vi "getAnalyisNuber.vi"(8 "Erreur en entrée":errorcluster caption="entrée d'erreur (pas d'erreur)", 9 "Nom de l'analyse en entrée":string, 11 "VISA resource en entrée":refnum<visa-resource-name>) -> (0 "error out":errorcluster caption="sortie d'erreur", 1 "Nom de l'analyse en sortie":string, 2 "Numéro de la\nprochaine analyse":i32, 3 "VISA resource en sortie":refnum<visa-resource-name>)   [LabVIEW 2019]
panel:
  out "Tableau":string[](array[string])
  out "Nom des fichiers":string[](array[string])
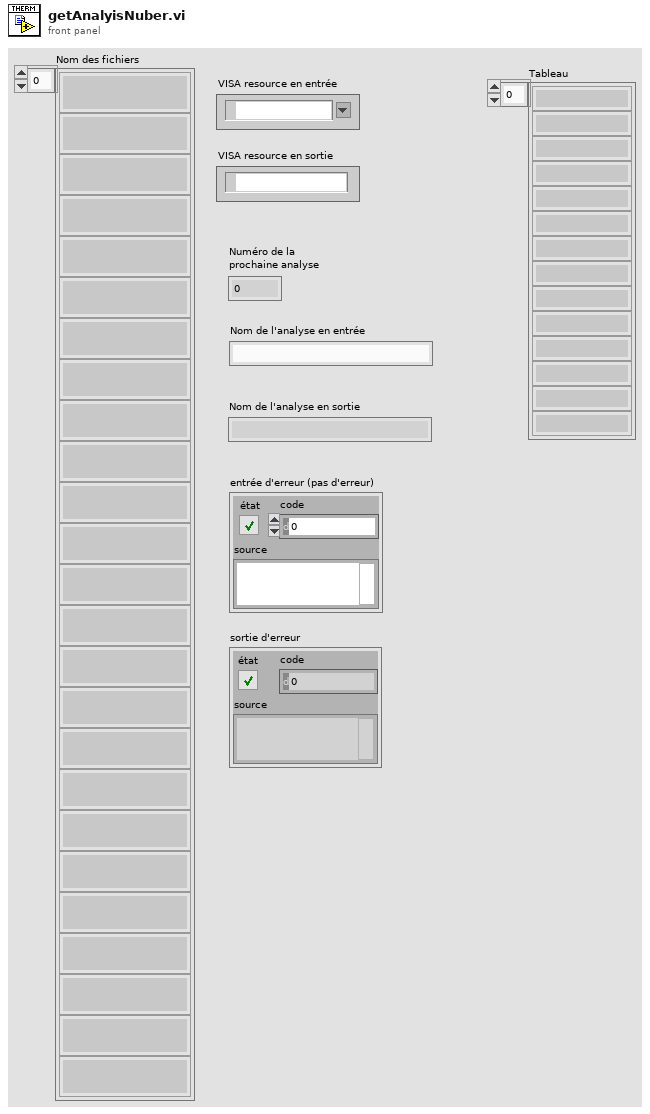
[diagram p1: front panel]
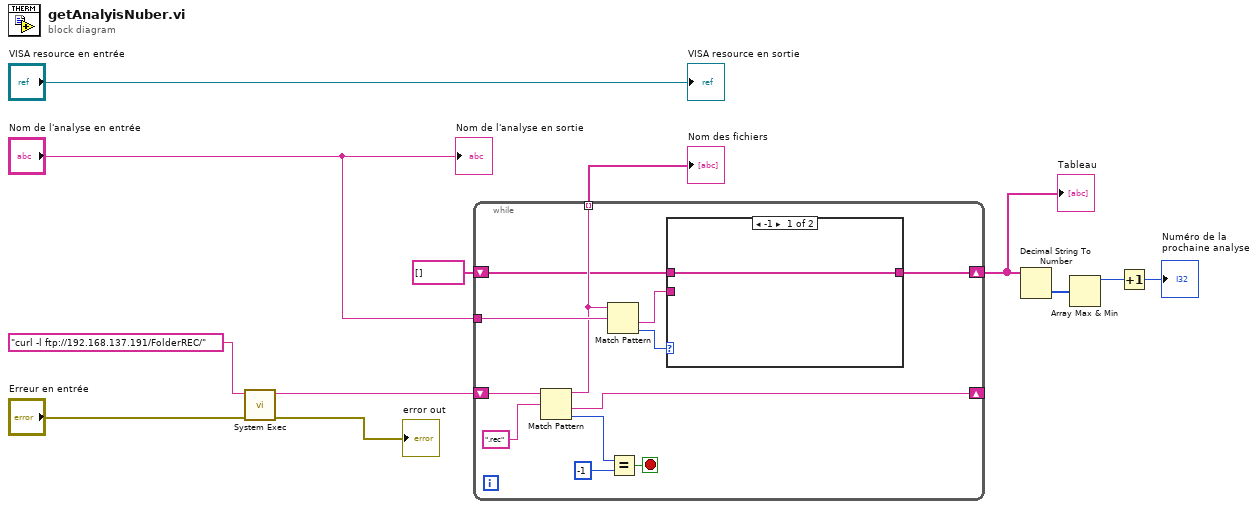
[diagram p0: block diagram]
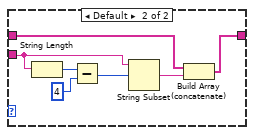
[diagram p2: hidden frame]
diagram:
  n1 = call <vilib>:"System Exec.vi"("error in (no error)"="Erreur en entrée", "command line"="curl -l ftp://192.168.137.191/FolderREC/") -> ("error out"=→"error out":errorcluster, "standard output"=w10:string)  [unwired: 6 in, 2 out]
  n2 = while {
    shift-right: [w20] -> _
    shift-left: w10 -> [w24]
    tunnel: [w18] -> w7 mode=indexing
    tunnel: "Nom de l'analyse en entrée" -> [w19]
    shift-right: [w17] -> w6
    shift-left: string[] [] -> [w16]
    stop <- w21 stop-if-true
    n3 = Match Pattern(string=w24, regular expression=".rec" ("expression régulière")) -> (before substring=w18:string, after substring=w20:string, offset past match=w23:i32)  [unwired: 1 in, 1 out]
    n4 = Match Pattern(string=w18, regular expression=w19) -> (after substring=w14:string, offset past match=w15:i32)  [unwired: 1 in, 2 out]
    n5 = Equal?(x=w23, y=-1) -> (x = y?=w21:bool)
    n6 = case shown="-1" w15 {
      tunnel: [w25 w32] -> w17
      tunnel: w14 -> [_ w27]
      tunnel: w16 -> [w25 w31]
      frame -1 {
      }
      frame Default {
        n7 = String Length(string=w27) -> (length=w29:i32)
        n8 = Subtract(x=w29, y=4) -> (x-y=w30:i32)
        n9 = String Subset(string=w27, offset (0)=w30) -> (substring=w26:string)  [unwired: 1 in]
        n10 = Build Array (concatenate)(w31, w26) -> (w32:string[])
      }
    }
  }
  "Nom des fichiers" <- w7
  "Tableau" <- w6
  n11 = Decimal String To Number(string=w6) -> (number=w5:i32[])  [unwired: 2 in, 1 out]
  n12 = Array Max & Min(array=w5) -> (max value=w4:i32)  [unwired: 3 out]
  n13 = Increment(x=w4) -> (x+1=→"Numéro de la\nprochaine analyse":i32)
  "VISA resource en sortie" <- "VISA resource en entrée"
  "Nom de l'analyse en sortie" <- "Nom de l'analyse en entrée"
